vi "ExecuteTestSuite.vi"   [LabVIEW 2010]
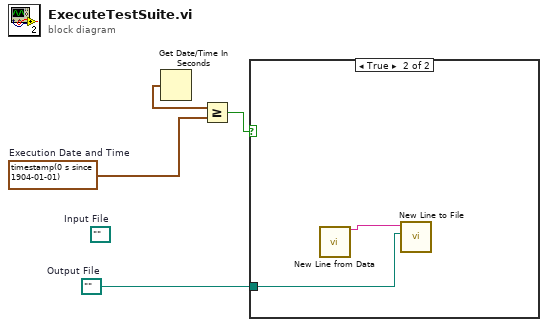
[diagram p0: block diagram]
diagram:
  (unwired) path ""  # Input File
  w1 = path ""  # Output File
  w3 = timestamp(0 s since 1904-01-01)  # Execution Date and Time
  n1 = Get Date/Time In Seconds() -> (seconds since 1Jan1904=w4:timestamp)
  n2 = Greater Or Equal?(x=w4, y=w3) -> (x >= y?=w2:bool)
  n3 = case shown="True" w2 {
    tunnel: w1 -> [_ w5]
    frame False {
    }
    frame True {
      n4 = call "New Line from Data.vi"() -> ("String"=w6:string)  [unwired: 19 in]
      n5 = call "New Line to File.vi"("Output File"=w5, "Text to add"=w6) -> ()  [unwired: 10 in]
    }
  }
